vi "Shutdown Device.vi"(8 "error in (no error)":errorcluster, 9 "01 Command? (F)":bool, 10 "Blast? (F)":bool, 11 "Serial Number":u32) -> (0 "error out":errorcluster, 3 "Tx array":u8[](array[numeric]))   [LabVIEW 2015]
uses:
  XceiverStates.ctl
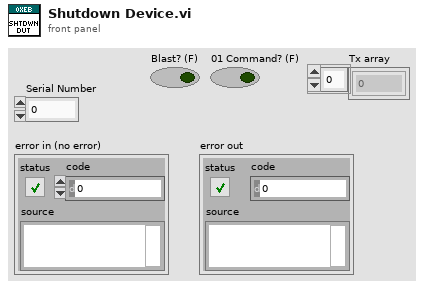
[diagram p1: front panel]
types:
  T1 = typedef "XceiverStates.ctl" = enum16{"Initialize", "Rx", "Tx", "Raw Mode", "Clear Buffer", "ClearEcho", "Read Buffer", "Close"}
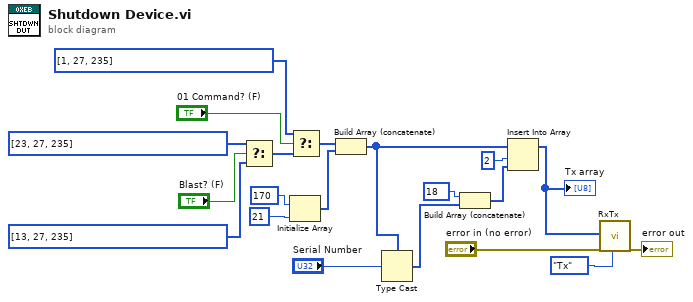
[diagram p0: block diagram]
diagram:
  n1 = Select(t=u8[] [23, 27, 235] ("initialized array"), s="Blast? (F)", f=u8[] [13, 27, 235] ("initialized array")) -> (s? t:f=w2:u8[])
  n2 = Initialize Array(u8 170, 21 ("dimension size")) -> (w12:u8[])
  n3 = Select(t=u8[] [1, 27, 235] ("initialized array"), s="01 Command? (F)", f=w2) -> (s? t:f=w1:u8[])
  n4 = Build Array (concatenate)(w1, w12) -> (w11:u8[])
  n5 = Type Cast(type=w11, x="Serial Number") -> (*(type *) &x=w13:u8[])
  n6 = Build Array (concatenate)(u8 18, w13) -> (w9:u8[])
  n7 = Insert Into Array(array=w11, index=2, new element=w9) -> (w20:u8[])
  "Tx array" <- w20
  n8 = call "RxTx.vi"("[TxData]"=w20, "error in (no error)"="error in (no error)", "Action"=XceiverStates."Tx") -> ("error out"=→"error out":errorcluster)  [unwired: 8 in, 8 out]
